vi "Unreserve Callback.vi"(8 "error in (no error)":errorcluster, 10 "session reservation":refnum<class "Session Reservation.lvclass">, 11 "reservation observer in":refnum<class "IReservationObserver.lvclass">) -> (0 "error out":errorcluster, 3 "reservation observer out":refnum<class "IReservationObserver.lvclass">)   [LabVIEW 2020, in "MeasurementLink Session Management.lvlib" / "IReservationObserver.lvclass"]
uses:
  IReservationObserver.lvclass
  Session Reservation/Session Reservation.lvclass
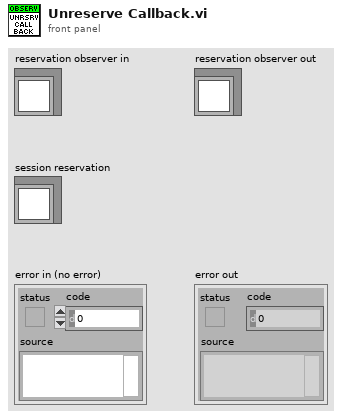
[diagram p1: front panel]
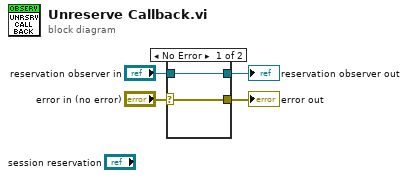
[diagram p0: block diagram]
diagram:
  n1 = case shown="No Error" "error in (no error)" {
    selector: "error in (no error)" -> [w5 w8]
    tunnel: [w5 w8] -> w3
    tunnel: [w6 w7] -> w1
    tunnel: "reservation observer in" -> [w6 w7]
    frame No Error {
    }
    frame Error {
    }
  }
  "error out" <- w3
  "reservation observer out" <- w1
